vi "test_Add Response.vi"(8 "error in (no error)":errorcluster, 11 "TestCase in":refnum<class "Instrument Addon Scripting API Messages Unit Tests.lvclass">) -> (0 "error out":errorcluster, 3 "TestCase out":refnum<class "Instrument Addon Scripting API Messages Unit Tests.lvclass">)   [LabVIEW 2018, in "Instrument Addon Scripting API Messages Unit Tests.lvclass"]
uses:
  Instrument Addon Scripting API Messages Unit Tests.lvclass
  APIs/Scripting API/TypeDefs/Wait Response Settings.ctl
  APIs/Scripting API/TypeDefs/Linked Channel.ctl
  <vilib>/NI Veristand/Custom Device API/Custom Device Item Ref.ctl
  NationalInstruments.VeriStand.SystemDefinitionAPI
  APIs/Scripting API/Messages/Add Response - Byte Count.vi
  <vilib>/addons/_JKI Toolkits/VI Tester/TestCase.llb/TestCase.lvclass
  Instrument Addon Scripting API Test Assets/Instrument Addon Scripting API Test Assets.lvclass
  APIs/Scripting API/Instrument Addon Scripting API.lvlib
  <vilib>/NI Veristand/Custom Device API/Custom Device API.lvlib
  C:/Program Files (x86)/National Instruments/LabVIEW 2018/vi.lib/addons/_JKI Toolkits/VI Tester/TestCase.llb/TestCase.lvclass
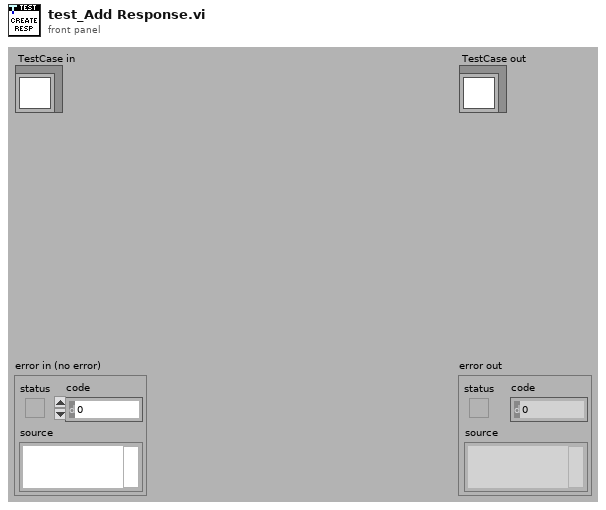
[diagram p1: front panel]
types:
  T1 = typedef "Custom Device API.lvlib/Custom Device Item Ref.ctl" = u64
  T2 = typedef "Instrument Addon Scripting API.lvlib/Linked Channel.ctl" = cluster{"Variable Name":string, "Channel Refnum":T1}
  T3 = typedef "Instrument Addon Scripting API.lvlib/Wait Response Settings.ctl" = cluster{"Response Format":string, "Linked Channels":T2[], "Byte Count":i32, "Use Byte Count channel":bool, "Channel Refnum":T1}
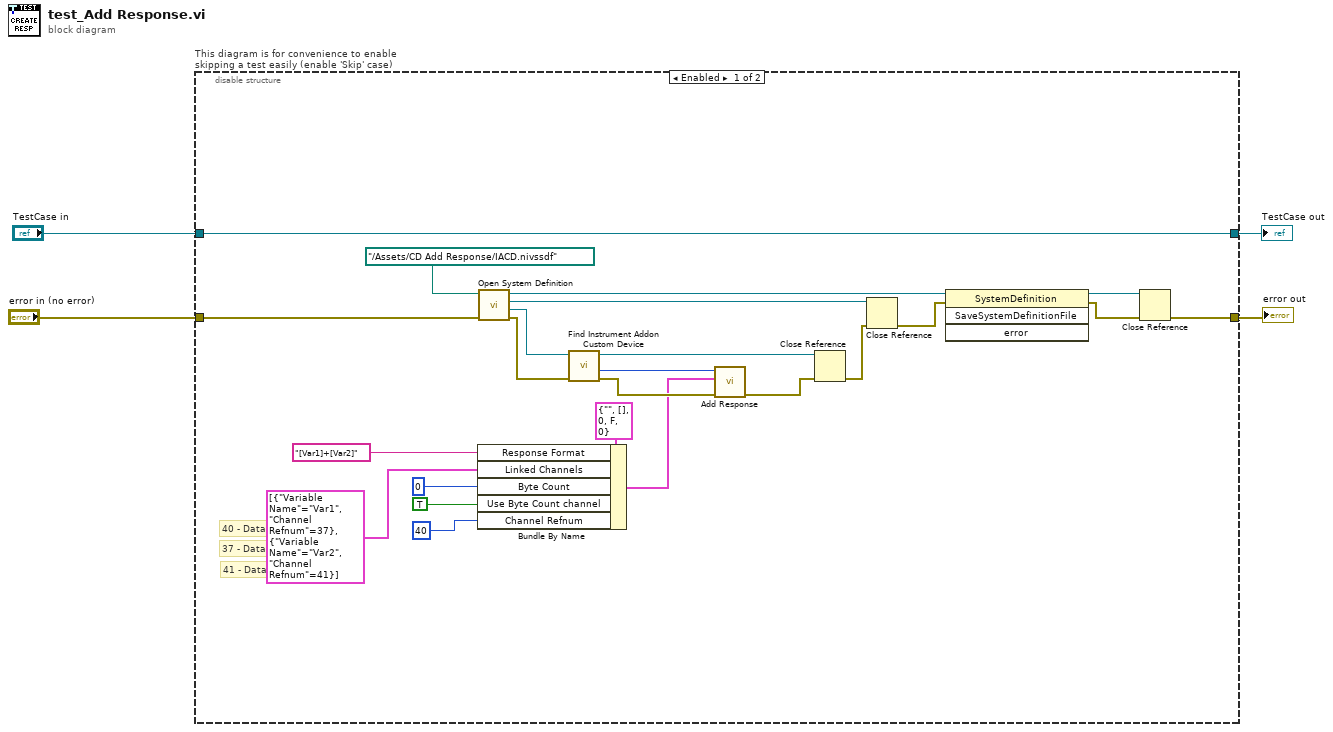
[diagram p0: block diagram]
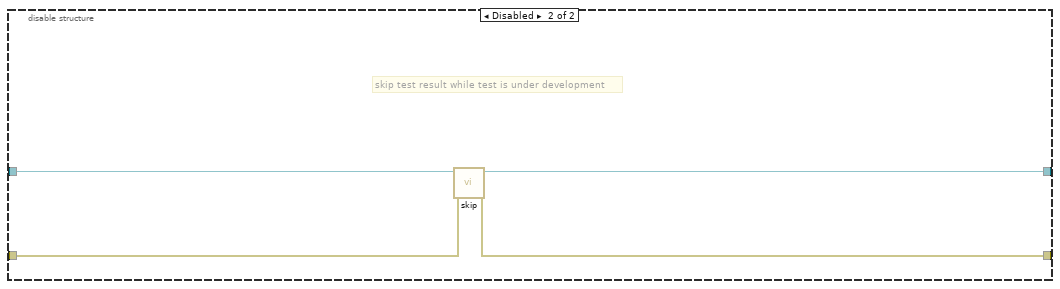
[diagram p2: hidden frame]
diagram:
  n1 = disable-structure "This diagram is for convenience to enable skipping a test easily (enable 'Skip' case)" shown="Enabled" {
    disable-tunnel: "TestCase in" -> [w20 w31]
    disable-tunnel: [w20 w29] -> w1
    disable-tunnel: [w21 w30] -> w3
    disable-tunnel: "error in (no error)" -> [w26 w28]
    frame Enabled {
      # "41 - Data 2"
      # "40 - Data 0"
      # "37 - Data 1"
      n2 = Bundle By Name(cluster=T3 {"Response Format"="", "Linked Channels"=[], "Byte Count"=0, "Use Byte Count channel"=FALSE, "Channel Refnum"=0} ("Settings"), "Response Format"="[Var1]+[Var2]", "Linked Channels"=T2[] [{"Variable Name"="Var1", "Channel Refnum"=37}, {"Variable Name"="Var2", "Channel Refnum"=41}], "Byte Count"=0, "Use Byte Count channel"=TRUE, "Channel Refnum"=T1 40) -> (w9:T3)
      n3 = call "Open System Definition.vi"("error in (no error)"=w26, "System Definition File"=path "../Assets/CD Add Response/IACD.nivssdf" ("SDF file")) -> ("error out"=w24:errorcluster, "Target Refnum"=w23:refnum<k24>, "Root Refnum"=w22:refnum<k24>, "System Definition Refnum"=w8:refnum<k24>)  [unwired: 6 in]
      n4 = call "Find Instrument Addon Custom Device.vi"("error in"=w24, "target in"=w23) -> ("error out"=w19:errorcluster, "NodeID"=w18:u64, "target out"=w16:refnum<k24>)  [unwired: 7 in]
      n5 = call-poly "Add Response.vi"("error in (no error)"=w19, "Settings"=w9, "Message in"=w18) -> ("error out"=w17:errorcluster)  [unwired: 7 in, 1 out]
      n6 = Close Reference(reference=w16, error in (no error)=w17) -> (error out=w25:errorcluster)
      n7 = Close Reference(reference=w22, error in (no error)=w25) -> (error out=w7:errorcluster)
      n8 = invoke class="SystemDefinition" method="SaveSystemDefinitionFile"(reference=w8, error in=w7) -> (reference out=w6:refnum<k24>, error out=w5:errorcluster)  [unwired: 2 in, 2 out]
      n9 = Close Reference(reference=w6, error in (no error)=w5) -> (error out=w21:errorcluster)
    }
    frame Disabled {
      # "skip test result while test is under development"
      n10 = call <vilib>:"skip.vi"("error in (no error)"=w28, "TestCase in"=w31) -> ("error out"=w30:errorcluster, "TestCase out"=w29:refnum<class "Instrument Addon Scripting API Messages Unit Tests.lvclass">)  [unwired: 8 in]
    }
  }
  "error out" <- w3
  "TestCase out" <- w1
